vi "Dummy UI.vi"() -> ()   [LabVIEW 2024]
panel:
  in  "Numeric":dbl
  in  "String":string
  out "Waveform Chart":dbl(graph)
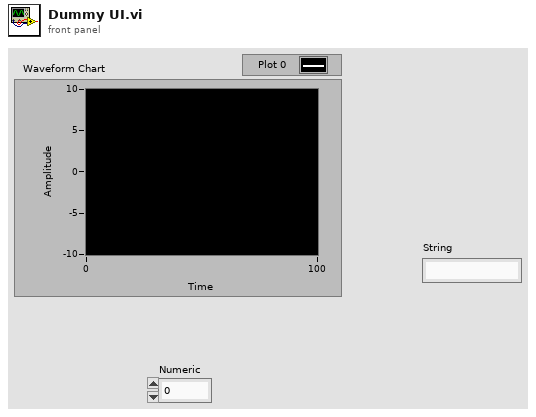
[diagram p1: front panel]
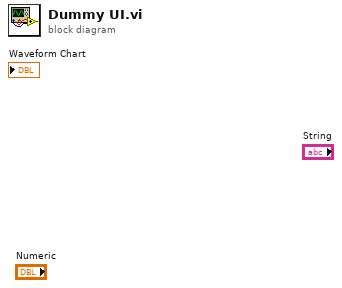
[diagram p0: block diagram]
diagram:
